vi "Read HttpContent.vi"(8 "error in (no error)":errorcluster, 11 "HttpRequestMessage in":refnum<class "HttpRequestMessage.lvclass">) -> (0 "error out":errorcluster, 2 "HttpContent":refnum<class "HttpContent.lvclass">, 3 "HttpRequestMessage out":refnum<class "HttpRequestMessage.lvclass">)   [LabVIEW 2018, in "HttpClient_NET.lvlib" / "HttpRequestMessage.lvclass"]
doc: "<b> </b> <b> </b>\nHttpClient_NET\nJustin Young - Viviota\nCopyright (c) 2021\nLicense: BSD"
uses:
  HttpRequestMessage.lvclass
  HttpContent/HttpContent.lvclass
  HttpRequestMessage.lvclass/HttpRequestMessage.ctl
  System.Net.Http
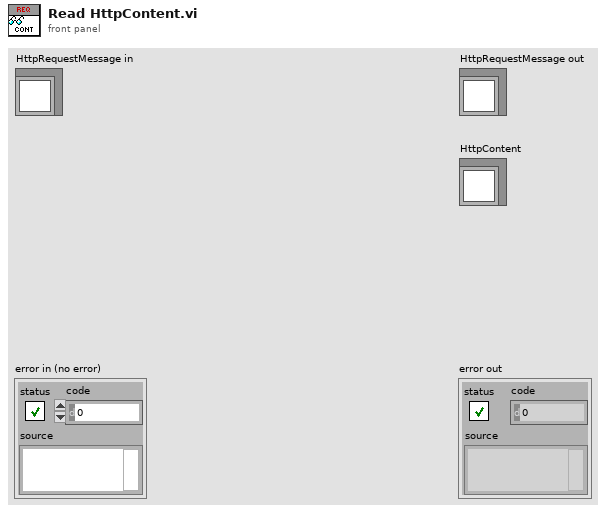
[diagram p1: front panel]
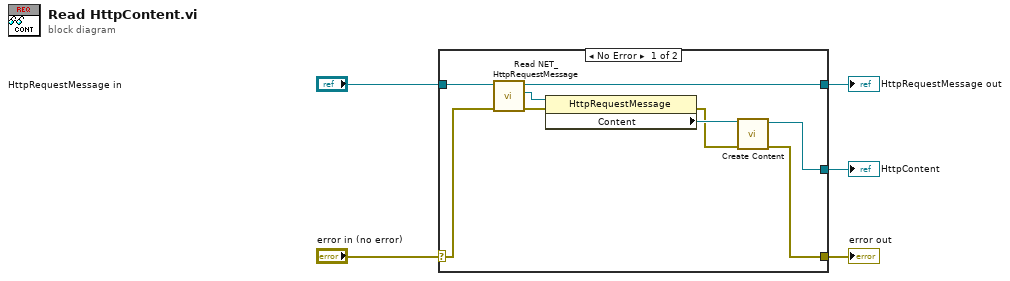
[diagram p0: block diagram]
diagram:
  n1 = case shown="No Error" "error in (no error)" {
    selector: "error in (no error)" -> [w13 w15]
    tunnel: [w6 w15] -> w4
    tunnel: [w8 w16] -> w2
    tunnel: "HttpRequestMessage in" -> [w14 w16]
    tunnel: [w9 _] -> w1
    frame No Error {
      n2 = call "Read NET_HttpRequestMessage.vi"("error in (no error)"=w13, "HttpRequestMessage in"=w14) -> ("error out"=w12:errorcluster, "NET_HttpRequestMessage"=w11:refnum<k24>, "HttpRequestMessage out"=w8:refnum<class "HttpRequestMessage.lvclass">)  [unwired: 7 in]
      n3 = property class="HttpRequestMessage"(reference=w11, error in=w12) -> (error out=w7:errorcluster, "Content"=w10:refnum<k24>)  [unwired: 1 out]
      n4 = call "Create Content.vi"("error in (no error)"=w7, "NET_HttpContent"=w10) -> ("error out"=w6:errorcluster, "HttpContent out"=w9:refnum<class "HttpContent.lvclass">)  [unwired: 8 in]
    }
    frame Error {
    }
  }
  "error out" <- w4
  "HttpRequestMessage out" <- w2
  "HttpContent" <- w1
